vi "Configure Output.vi"(7 "Enable Channel Output (F: False)":bool, 8 "error in (no error)":errorcluster, 9 "Voltage Level (0.0 V)":dbl format="%.3g", 10 "Channel (1:1)":u16(ring)=1 items=["1"=1, "2"=2, "3"=3], 11 "VISA resource name":refnum<visa-resource-name>) -> (0 "error out":errorcluster, 3 "VISA resource name out":refnum<visa-resource-name>)   [LabVIEW 2017, in "BK Precision 913XX.lvlib"]
doc: "Configures output voltage level output and output state of the selected channel."
uses:
  <instrlib>/BK Precision 913XX/BK Precision 913XX.lvlib
panel:
  # "V"
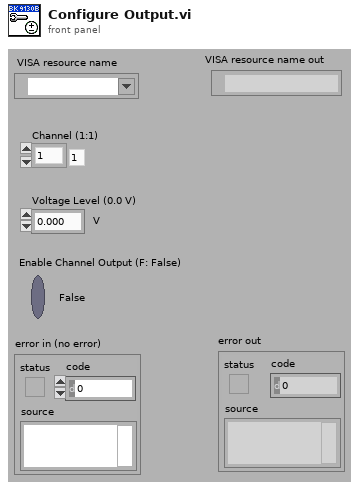
[diagram p1: front panel]
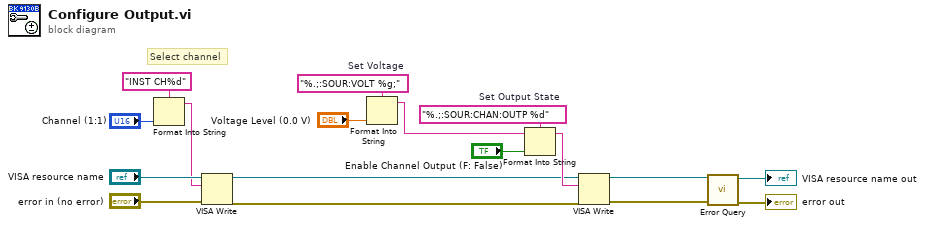
[diagram p0: block diagram]
diagram:
  w13 = "%.;:SOUR:CHAN:OUTP %d"  # Set Output State
  w15 = "%.;:SOUR:VOLT %g;"  # Set Voltage
  # "Select channel"
  n1 = Format Into String(format string="INST CH%d", "Channel (1:1)") -> (resulting string=w3:string)  [unwired: 2 in, 1 out]
  n2 = VISA Write(VISA resource name="VISA resource name", write buffer=w3, error in (no error)="error in (no error)") -> (VISA resource name out=w8:refnum<visa-resource-name>, error out=w7:errorcluster)  [unwired: 1 out]
  n3 = Format Into String(format string=w15, "Voltage Level (0.0 V)") -> (resulting string=w6:string)  [unwired: 2 in, 1 out]
  n4 = Format Into String(format string=w13, initial string=w6, "Enable Channel Output (F: False)") -> (resulting string=w11:string)  [unwired: 1 in, 1 out]
  n5 = VISA Write(VISA resource name=w8, write buffer=w11, error in (no error)=w7) -> (VISA resource name out=w1:refnum<visa-resource-name>, error out=w2:errorcluster)  [unwired: 1 out]
  n6 = call <instrlib>:"Error Query.vi"("error in (no error)"=w2, "VISA resource name"=w1) -> ("error out"=→"error out":errorcluster, "VISA resource name out"=→"VISA resource name out":refnum<visa-resource-name>)  [unwired: 6 in, 2 out]
